vi "init text report (SubVI).vi"(8 "error in (no error)":errorcluster, 10 "String to file":string="This is the content", 11 "Serial Number":string="34643634.txt") -> (0 "error out":errorcluster, 3 "refnum out":refnum<file>)   [LabVIEW 2013]
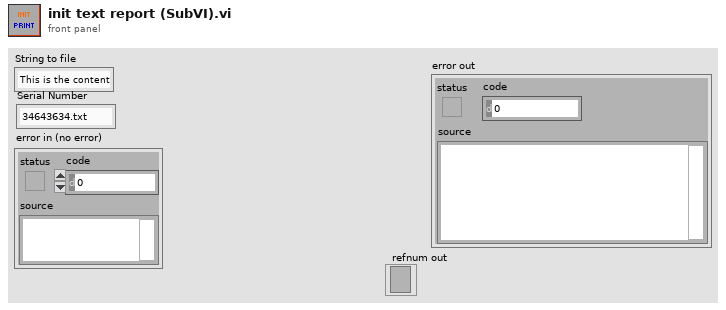
[diagram p1: front panel]
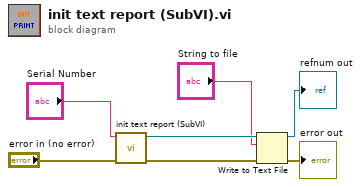
[diagram p0: block diagram]
diagram:
  n1 = call "init text report (SubVI).vi"("error in (no error)"="error in (no error)", "Serial Number"="Serial Number") -> ("error out"=w6:errorcluster, "refnum out"=w5:refnum<file>)  [unwired: 8 in]
  n2 = Write to Text File(file (use dialog)=w5, text="String to file", error in=w6) -> (refnum out=→"refnum out":refnum<file>, error out=→"error out":errorcluster)  [unwired: 1 in, 1 out]
